vi "Read Command Sequence File.vi"(11 "Path Name":string) -> (3 "Auto Commands":T1=[{"Drive Duration"=0.0, "Left Speed"=0.0, "Right Speed"=0.0, "Set Point"=1.0, "Set Point Duration"=2.0, "Command"=enum."Shooter", "Wait ms"=0.0}, {"Drive Duration"=0.0, "Left Speed"=0.0, "Right Speed"=0.0, "Set Point"=0.0, "Set Point Duration"=0.0, "Command"=enum."Wait", "Wait ms"=100.0}, {"Drive Duration"=0.0, "Left Speed"=0.0, "Right Speed"=0.0, "Set Point"=0.5, "Set Point Duration"=2.0, "Command"=enum."Transfer", "Wait ms"=0.0}])   [LabVIEW 2019]
uses:
  Controls/Auto Controls.ctl
  Controls/Command Sequene single Control.ctl
  <vilib>/Utility/file.llb/Read Delimited Spreadsheet (DBL).vi
panel:
  out "all rows 2":dbl[](array[numeric])
  out "all rows":dbl[][](array[numeric])
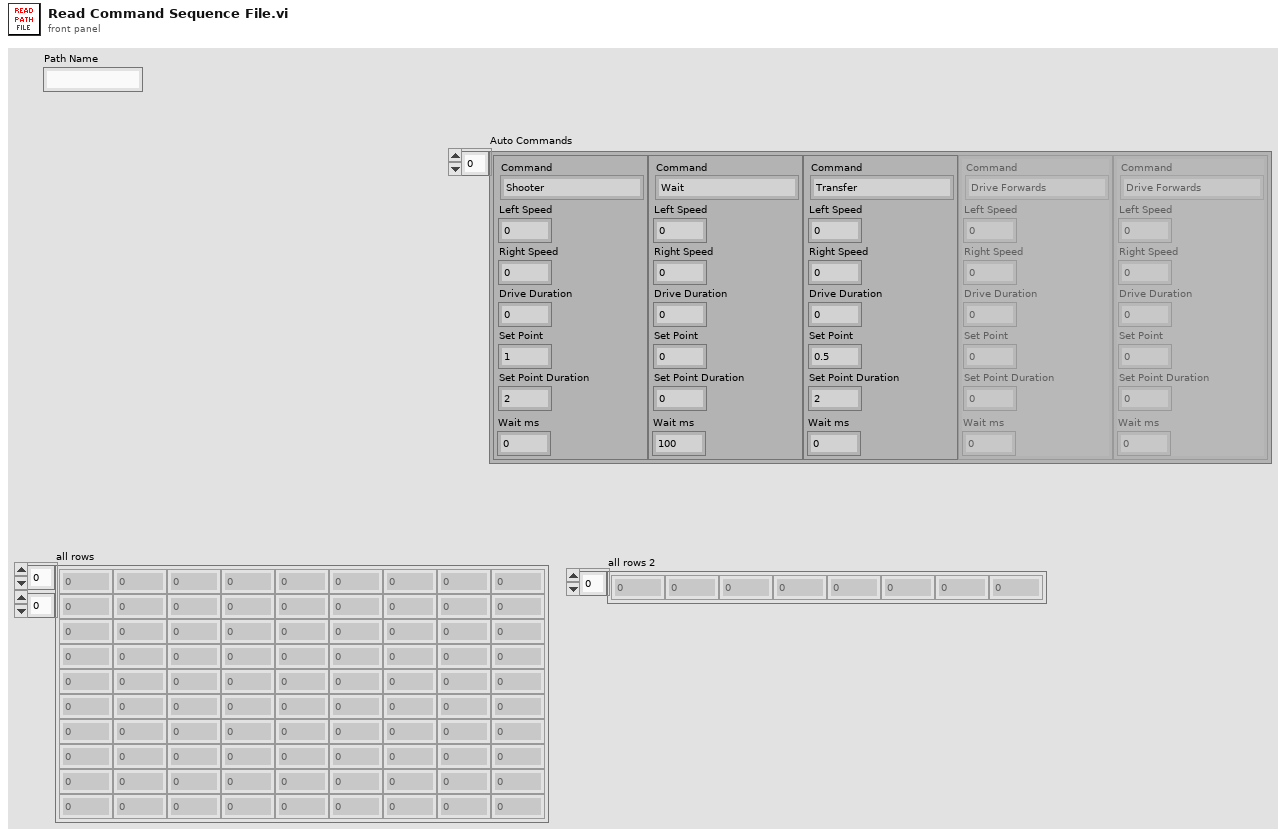
[diagram p1: front panel]
types:
  T1 = typedef "Auto Controls.ctl" = cluster{"Drive Duration":dbl, "Left Speed":dbl, "Right Speed":dbl, "Set Point":dbl, "Set Point Duration":dbl, "Command":enum16{"", "Drive Forwards", "Drive Backwards", "Stop", "Turn Left", "Turn Right", "Drop Intake", "Lift Intake", "Intake", "Shooter", "Transfer", "Wait"}, "Wait ms":dbl}[]
  T2 = typedef "Command Sequene single Control.ctl" = cluster{"Drive Duration":dbl, "Left Speed":dbl, "Right Speed":dbl, "Set Point":dbl, "Set Point Duration":dbl, "Command":enum16{"", "Drive Forwards", "Drive Backwards", "Stop", "Turn Left", "Turn Right", "Drop Intake", "Lift Intake", "Intake", "Shooter", "Transfer", "Wait"}, "Wait ms":dbl}
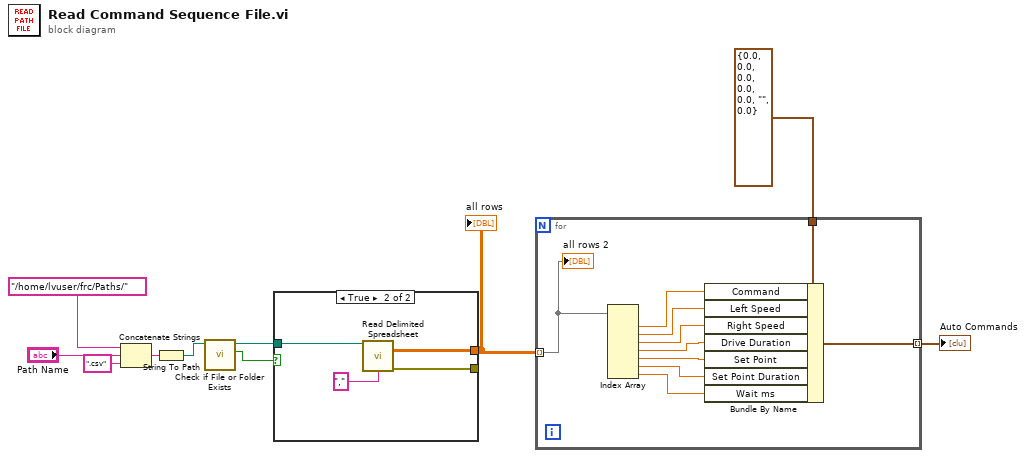
[diagram p0: block diagram]
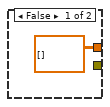
[diagram p2: hidden frame]
diagram:
  n1 = Concatenate Strings("/home/lvuser/frc/Paths/" ("string"), "Path Name", ".csv" ("string")) -> (w4:string)
  n2 = String To Path(string=w4) -> (path=w3:path)
  n3 = call <vilib>:"Check if File or Folder Exists.vi"("path"=w3) -> ("file or folder exists?"=w8:bool, "dup path"=w7:path)  [unwired: 8 in, 1 out]
  n4 = case shown="True" w8 {
    tunnel: w7 -> [_ w15]
    tunnel: [dbl[][] [] ("all rows") w14] -> w6
    tunnel: [_ w12] -> _
    frame False {
    }
    frame True {
      n5 = call-poly <vilib>:"Read Delimited Spreadsheet.vi"("file path (dialog if empty)"=w15, "delimiter (\\t)"="," ("delimiter (\\t)")) -> ("all rows"=w14:dbl[][], "error out"=w12:errorcluster)  [unwired: 8 in, 4 out]
    }
  }
  "all rows" <- w6
  n6 = for {
    tunnel: w6 -> [w24] mode=indexing
    tunnel: T2 {"Drive Duration"=0.0, "Left Speed"=0.0, "Right Speed"=0.0, "Set Point"=0.0, "Set Point Duration"=0.0, "Command"=enum."", "Wait ms"=0.0} ("Auto Control") -> [w25]
    tunnel: [w16] -> w1 mode=indexing
    n7 = Index Array(array=w24) -> (element #1=w23:dbl, element #2=w22:dbl, element #3=w21:dbl, element #4=w20:dbl, element #5=w19:dbl, element #6=w18:dbl, element #7=w17:dbl)  [unwired: 7 in]
    n8 = Bundle By Name(cluster=w25, "Command"=w23, "Left Speed"=w22, "Right Speed"=w21, "Drive Duration"=w20, "Set Point"=w19, "Set Point Duration"=w18, "Wait ms"=w17) -> (w16:T2)
    "all rows 2" <- w24
  }
  "Auto Commands" <- w1
